vi "Web receiver.vi"(11 "queue in":refnum<queue>) -> (2 "Connected?":bool, 3 "Device trying to connect":bool)   [LabVIEW 2014]
uses:
  controls/UI Data.ctl
  controls/Web command parser enum.ctl
  controls/UI DataSam.ctl
  globals/RT Network Stream Endpoints.vi
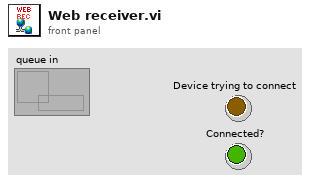
[diagram p1: front panel]
types:
  T1 = typedef "Web command parser enum.ctl" = enum16{"Wait for connect", "Write Commands"}
  T2 = typedef "UI DataSam.ctl" = cluster{"Message":string, "Data":variant}
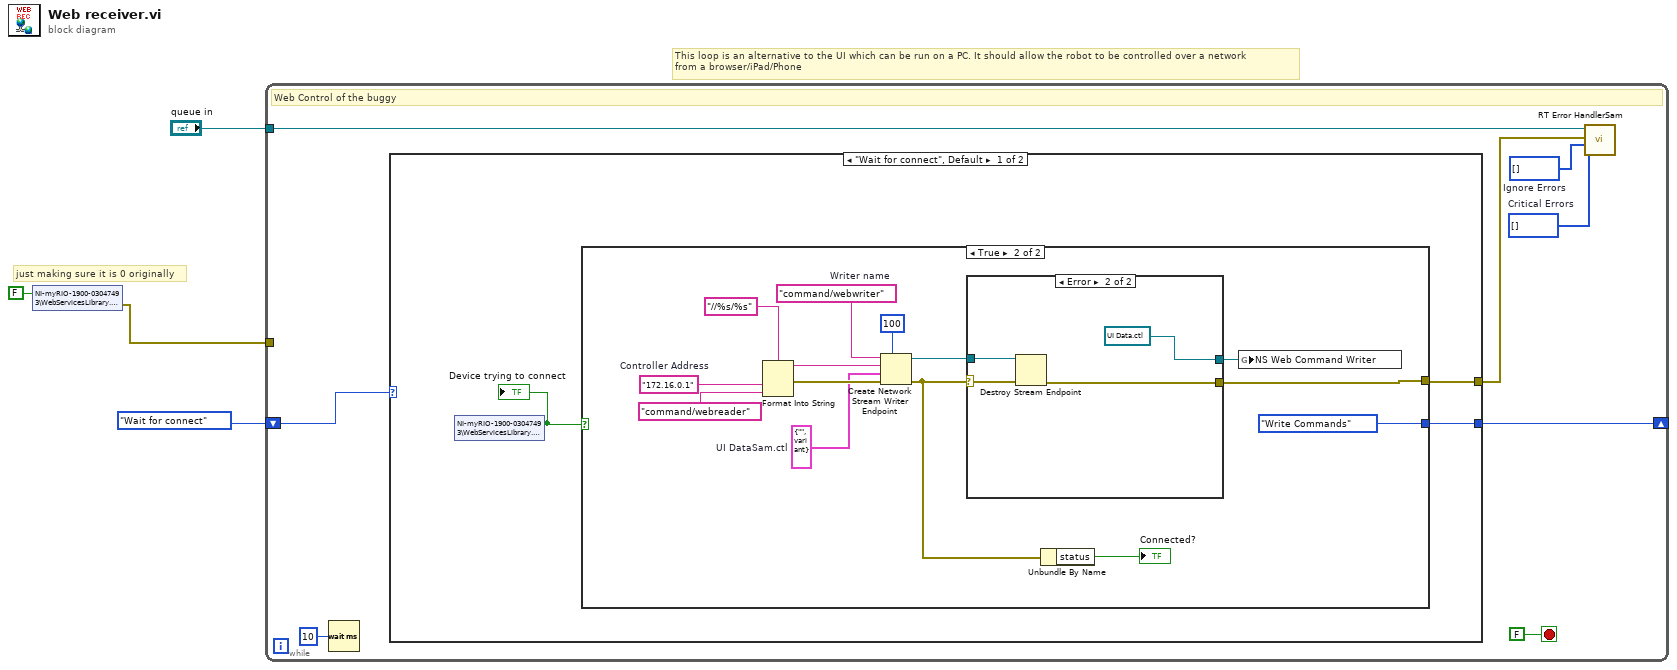
[diagram p0: block diagram]
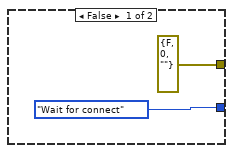
[diagram p2: hidden frame]
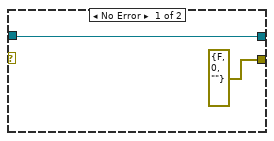
[diagram p3: hidden frame]
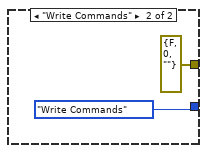
[diagram p4: hidden frame]
diagram:
  # "just making sure it is 0 originally"
  # "This loop is an alternative to the UI which can be run on a PC. It should allow the robot to be controlled over a network\nfrom a browser/iPad/Phone"
  n1 = shared-variable "NI-myRIO-1900-03047493\\WebServicesLibrary.lvlib\\Connect"(FALSE ("Connect")) -> (error out=w1:errorcluster)  [unwired: 1 in]
  n2 = while {
    tunnel: "queue in" -> [w9]
    shift-right: [w6] -> _
    shift-left: Web_command_parser_enum."Wait for connect" ("Command Parser Enum") -> [w5]
    tunnel: w1 -> [_]
    stop <- FALSE stop-if-true
    w10 = i32[] []  # Ignore Errors
    w11 = i32[] []  # Critical Errors
    # "Web Control of the buggy"
    n3 = Wait (ms)(milliseconds to wait=u32 10) -> ()  [unwired: 1 out]
    n4 = case shown="\"Wait for connect\", Default" w5 {
      tunnel: [w15 errorcluster {"status"=FALSE, "code"=0, "source"=""} ("error out")] -> w8
      tunnel: [w13 Web_command_parser_enum."Write Commands" ("Command Parser Enum")] -> w6
      frame "Wait for connect", Default {
        n5 = shared-variable "NI-myRIO-1900-03047493\\WebServicesLibrary.lvlib\\Connect"() -> (w14:bool)  [unwired: 1 in, 1 out]
        "Device trying to connect" <- w14
        n6 = case shown="True" w14 {
          tunnel: [errorcluster {"status"=FALSE, "code"=0, "source"=""} ("error out") w22] -> w15
          tunnel: [Web_command_parser_enum."Wait for connect" ("Command Parser Enum") Web_command_parser_enum."Write Commands" ("Command Parser Enum")] -> w13
          frame False {
          }
          frame True {
            w21 = "172.16.0.1"  # Controller Address
            w25 = T2 {"Message"="", "Data"=variant}  # UI DataSam.ctl
            w26 = "command/webwriter"  # Writer name
            n7 = Format Into String(format string="//%s/%s", w21, "command/webreader" ("input 2")) -> (resulting string=w28:string, error out=w29:errorcluster)  [unwired: 2 in]
            n8 = Create Network Stream Writer Endpoint(7:100 ("writer buffer size"), 8:w29, 9:w25, 10:w28, 11:w26) -> (0:w23:errorcluster, 3:w24:refnum<k21>)  [unwired: 2 in]
            n9 = case shown="Error" w23 {
              selector: w23 -> [_ w37]
              tunnel: w24 -> [w33 w36]
              tunnel: [w33 refnum<k21> refnum ("Writer name")] -> w18
              tunnel: [errorcluster {"status"=FALSE, "code"=0, "source"=""} ("error out") w34] -> w22
              frame No Error {
              }
              frame Error {
                n10 = Destroy Stream Endpoint(8:w37, 11:w36) -> (0:w34:errorcluster)
              }
            }
            n11 = Unbundle By Name(w23) -> ("status"=→"Connected?":bool)
            n12 = global write "RT Network Stream Endpoints.vi" "NS Web Command Writer"(w18) -> ()
          }
        }
      }
      frame "Write Commands" {
      }
    }
    n13 = call "RT Error HandlerSam.vi"("Ignore Errors"=w10, "Critical Errors"=w11, "error to process"=w8, "queue in"=w9) -> ()  [unwired: 7 in, 1 out]
  }
